vi "Append VI Description to Report (path).vi"(0 "report in":refnum<class "NI_report.lvclass">, 5 "VI":path, 11 "error in (no error)":errorcluster, 12 "MS Office parameters":T1) -> (4 "report out":refnum<class "NI_report.lvclass">, 6 "VI path out":path, 8 "start out (Word)":i32, 10 "end out (Word)":i32, 15 "error out":errorcluster)   [LabVIEW 2020, in "NI_ReportGenerationCore.lvlib"]
doc: "Appends the description of the VI you specify in <B>VI</B> to a report. Wire data to the <B>VI</B> input to determine the polymorphic instance to use or manually select the instance."
uses:
  <vilib>/Utility/NIReport.llb/NI_ReportGenerationCore.lvlib
  <vilib>/Utility/NIReport.llb/NI_report.lvclass
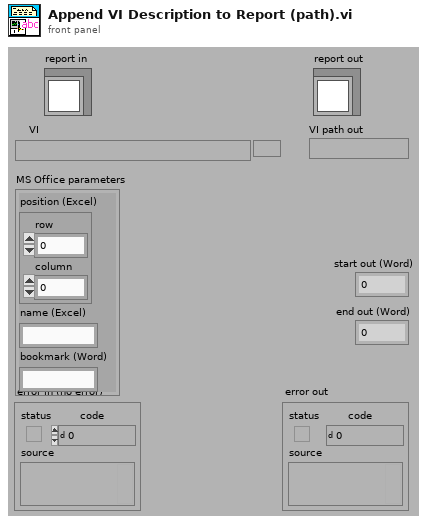
[diagram p1: front panel]
types:
  T1 = cluster{"position (Excel)":cluster{"row":i32, "column":i32}, "name (Excel)":string, "bookmark (Word)":string}
  T2 = enum32{"invalid app kind", "Development System", "Run Time System", "Student Edition", "Embedded LabVIEW", "Evaluation", "Custom"}
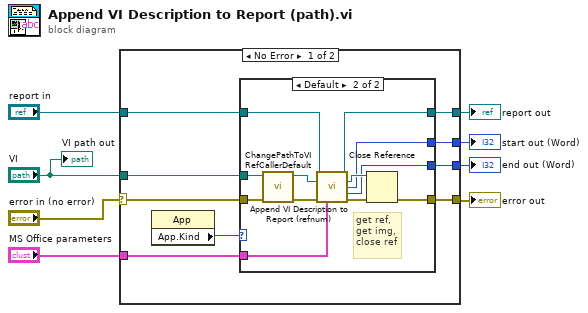
[diagram p0: block diagram]
diagram:
  n1 = case shown="No Error" "error in (no error)" {
    selector: "error in (no error)" -> [w15 w33]
    tunnel: [w13 w33] -> w7
    tunnel: [w16 w32] -> w5
    tunnel: "report in" -> [w17 w32]
    tunnel: "VI" -> [w10 _]
    tunnel: "MS Office parameters" -> [w14 _]
    tunnel: [w12 _] -> w2
    tunnel: [w11 _] -> w1
    frame No Error {
      n2 = property class="App"() -> ("App.Kind"=w9:T2)  [unwired: 2 in, 2 out]
      n3 = case shown="Default" w9 {
        tunnel: w17 -> [w19 w31]
        tunnel: [w19 w21] -> w16
        tunnel: w15 -> [w18 w30]
        tunnel: w14 -> [_ w28]
        tunnel: [w18 w25] -> w13
        tunnel: [_ w24] -> w12
        tunnel: [_ w20] -> w11
        tunnel: w10 -> [_ w22]
        frame "Run Time System" {
          # "Do not try to append\nif running in an\nexecutable"
        }
        frame Default {
          # "get ref,\nget img,\nclose ref"
          n4 = call <vilib>:"ChangePathToVIRefCallerDefault.vi"("error in (no error)"=w30, "VI path"=w22) -> ("error out"=w29:errorcluster, "VI reference"=w23:refnum<vi>)  [unwired: 4 in]
          n5 = call <vilib>:"Append VI Description to Report (refnum).vi"("report in"=w31, "VI"=w23, "error in (no error)"=w29, "MS Office parameters"=w28) -> ("report out"=w21:refnum<class "NI_report.lvclass">, "VI out"=w27:refnum<vi>, "start out (Word)"=w24:i32, "end out (Word)"=w20:i32, "error out"=w26:errorcluster)  [unwired: 7 in]
          n6 = Close Reference(reference=w27, error in (no error)=w26) -> (error out=w25:errorcluster)
        }
      }
    }
    frame Error {
    }
  }
  "error out" <- w7
  "report out" <- w5
  "start out (Word)" <- w2
  "end out (Word)" <- w1
  "VI path out" <- "VI"
